vi "getData.vi"(8 "error in (no error)":errorcluster, 11 "reference in":refnum<class "Devices Controller.lvclass">) -> (0 "error out":errorcluster, 2 "data":string[][][](array[string]), 3 "reference out":refnum<class "Devices Controller.lvclass">)   [LabVIEW 2015, in "Devices Controller.lvclass"]
uses:
  Devices Controller.lvclass
  APP/excelFile_class/fileType.ctl
  File Controller_llb/File Controller.lvclass
  APP/excelFile_class/excelFile.lvclass
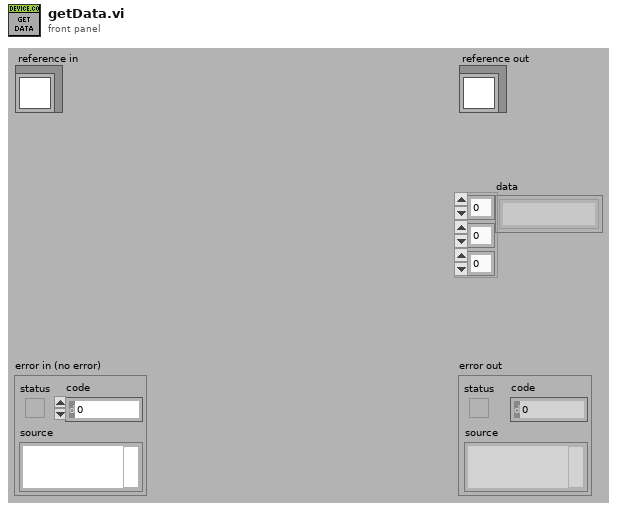
[diagram p1: front panel]
types:
  T1 = typedef "excelFile.lvclass/fileType.ctl" = enum16{"devices", "items", "partsTracking"}
  T2 = typedef "Devices Controller.lvclass/ObjectAttributesRef.ctl" = refnum<data-value>
  T3 = typedef "Devices Controller.lvclass/ObjectAttributes.ctl" = cluster{"MyAttribute":dbl, "file_controller_ref":refnum<class "File Controller.lvclass">, "data":string[][][], "devices_refs":cluster{"k4b2_refs":refnum<class "k4b2.lvclass">[], "rmr_refs":refnum<class "rmr.lvclass">[], "bod_pod_refs":refnum<class "bodpod.lvclass">[], "cpet_refs":refnum<class "cpet.lvclass">[], "fitmate_refs":refnum<class "fitmate.lvclass">[], "pea_pod_refs":refnum<class "peapod.lvclass">[], "k5_refs":refnum<class "k5.lvclass">[], "bb-pft_refs":refnum<class "bb-pft.lvclass">[]}}
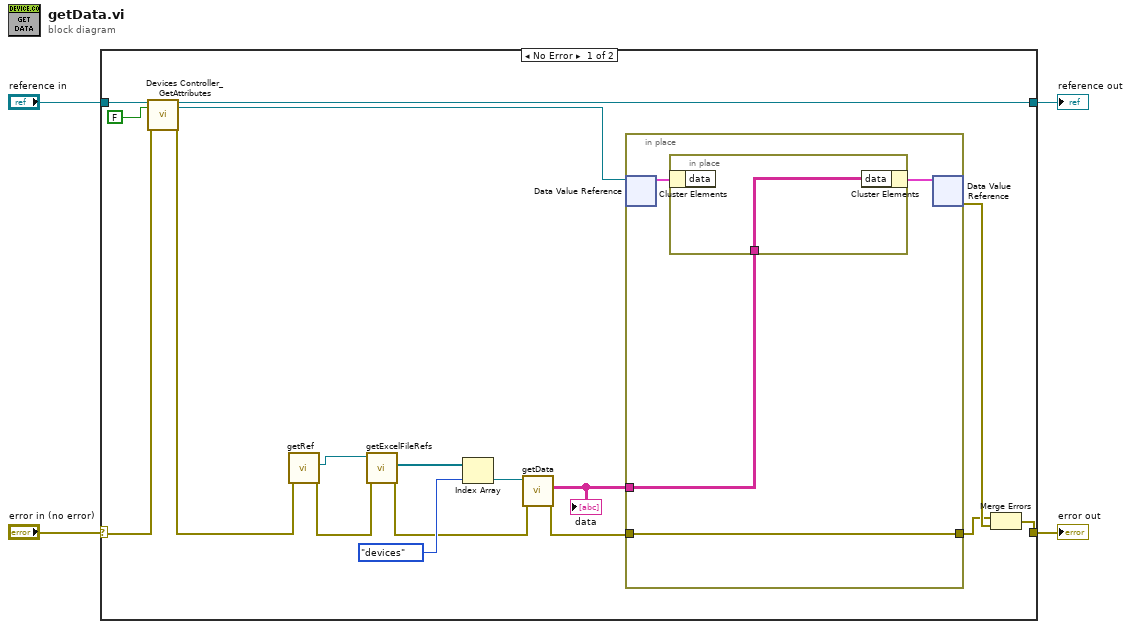
[diagram p0: block diagram]
diagram:
  n1 = case shown="No Error" "error in (no error)" {
    selector: "error in (no error)" -> [w16 w28]
    tunnel: [w21 w28] -> w3
    tunnel: [w15 w27] -> w1
    tunnel: "reference in" -> [w18 w27]
    frame No Error {
      n2 = call "Devices Controller_GetAttributes.vi"("reference in"=w18, "return data? (T)"=FALSE, "error in (no error)"=w16) -> ("reference out"=w15:refnum<class "Devices Controller.lvclass">, "attributes ref"=w14:T2, "error out"=w7:errorcluster)  [unwired: 13 in, 1 out]
      n3 = call "getRef.vi"("error in (no error)"=w7) -> ("error out"=w12:errorcluster, "File Controller_ref"=w13:refnum<class "File Controller.lvclass">)  [unwired: 9 in]
      n4 = call "getExcelFileRefs.vi"("error in (no error)"=w12, "reference in"=w13) -> ("error out"=w9:errorcluster, "excelFile_refs"=w11:refnum<class "excelFile.lvclass">[])  [unwired: 7 in, 1 out]
      n5 = Index Array(array=w11, index=fileType."devices" ("fileType")) -> (element=w8:refnum<class "excelFile.lvclass">)
      n6 = call "getData.vi"("error in (no error)"=w9, "reference in"=w8) -> ("error out"=w6:errorcluster, "data"=w5:string[][][])  [unwired: 7 in, 1 out]
      "data" <- w5
      n7 = in-place {
        in-place-border: w6 -> [w23]
        in-place-border: [w23] -> w19
        in-place-border: w5 -> [w22]
        n8 = in-place-dvr #1(w14) -> (w24:T3)  [unwired: 1 out]
        n9 = in-place {
          in-place-border: w22 -> [w26]
          n10 = in-place-cluster #2(w24) -> ()  [unwired: 1 out]
          n11 = in-place-cluster #2("data"=w26) -> (w25:T3)
        }
        n12 = in-place-dvr #1(w25) -> (w20:errorcluster)  [unwired: 1 out]
      }
      n13 = Merge Errors(w19, w20) -> (w21:errorcluster)
    }
    frame Error {
    }
  }
  "error out" <- w3
  "reference out" <- w1
